vi "Convert_CameraAngle_to_Distance.vi"(8 "a2":dbl, 9 "a1":dbl, 10 "h2":dbl, 11 "h1":dbl) -> (3 "d":dbl)   [LabVIEW 2019]
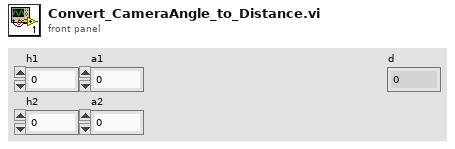
[diagram p1: front panel]
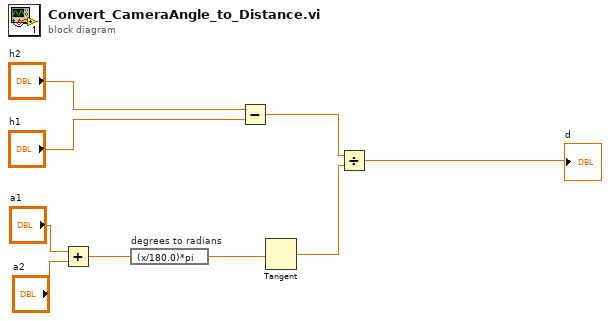
[diagram p0: block diagram]
diagram:
  n1 = Add(x="a1", y="a2") -> (x+y=w2:dbl)
  n2 = expression code="(x/180.0)*pi" "degrees to radians"(w2) -> (w1:dbl)
  n3 = Subtract(x="h2", y="h1") -> (x-y=w4:dbl)
  n4 = Tangent(1:w1) -> (0:w3:dbl)
  n5 = Divide(x=w4, y=w3) -> (x/y=→"d":dbl)
